vi "Otto_Stephen.vi"() -> ()   [LabVIEW 2020]
uses:
  <vilib>/MakerHub/LINX/Public/Peripherals/Analog/Analog Read 1 Chan.vi
  <vilib>/MakerHub/LINX/Public/Peripherals/Analog/Analog Read N Chans.vi
  <vilib>/MakerHub/LINX/Private/Local IO/LinxAnalogRead.vi
  <vilib>/MakerHub/LINX/Public/Utilities/Check Channel.vi
  <vilib>/MakerHub/LINX/Public/Utilities/Open Serial.vi
  <vilib>/MakerHub/LINX/Private/Utilties/Generate Error.vi
  <vilib>/MakerHub/LINX/LMH-LINX.lvlib
panel:
  out "Light":bool
  out "Voltage":dbl
  out "Waveform Chart":cluster{dbl, "f":dbl}(graph)
  in  "Offset":dbl
  in  "?":bool
  in  "Serial Port":refnum<visa-resource-name>="N/A"
  # "Stephen Otto\n011796499"
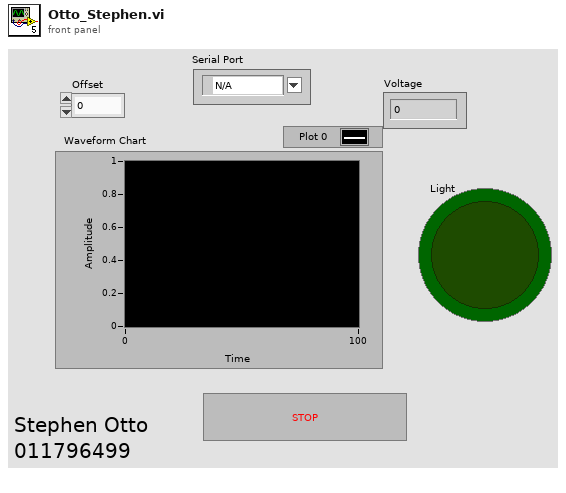
[diagram p1: front panel]
types:
  T1 = typedef "LMH-LINX.lvlib/LINX Ref.ctl" = cluster{"IO":T2, "Interface":T3, "LINX Device Config":T4}
  T2 = typedef "LMH-LINX.lvlib/Platform.ctl" = enum16{"Remote", "Local"}
  T3 = typedef "LMH-LINX.lvlib/Interface.ctl" = enum16{"Serial", "TCP"}
  T4 = typedef "LMH-LINX.lvlib/Device.lvlib/LINX Device Config.ctl" = cluster{"Interface":T3, "COM Port":refnum<visa-resource-name>, "TCP Configuration":T5, "Device Family":u8, "Device ID":u8, "Device Name":string, "TCP Ref":refnum<k5>, "Channels":T6}
  T5 = typedef "LMH-LINX.lvlib/Device.lvlib/TCP Config.ctl" = cluster{"IP Address":string, "Port":u16}
  T6 = typedef "LMH-LINX.lvlib/Channels.ctl" = cluster{"DI":u8[], "DO":u8[], "AI":u8[], "AO":u8[], "PWM":u8[], "QE":u8[], "UART":u8[], "I2C 2":u8[], "SPI":u8[], "CAN":u8[], "Servo":u8[], "AI Ref (V)":dbl, "AI Resolution (Bits)":u8, "AO Ref (V)":dbl, "AO Resolution (Bits)":u8}
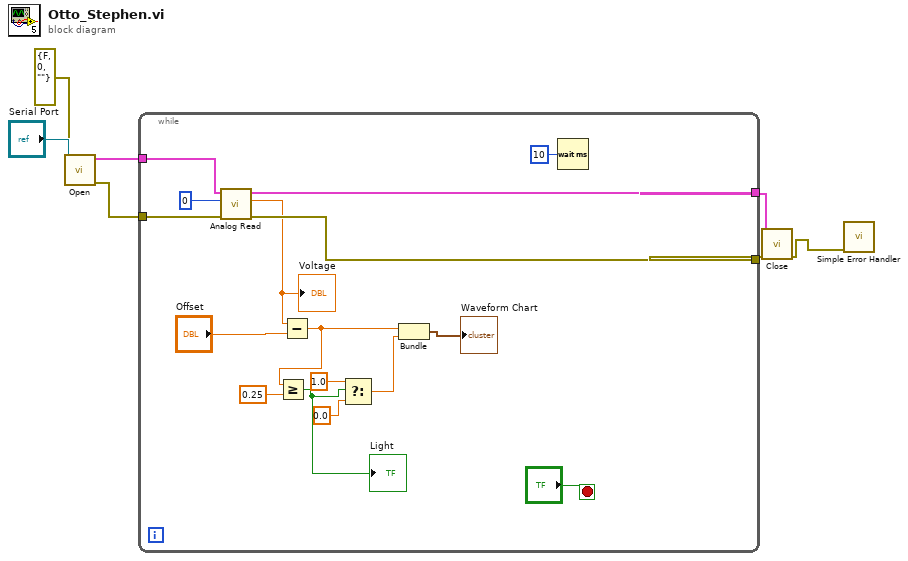
[diagram p0: block diagram]
diagram:
  n1 = call-poly <vilib>:"Open.vi"("Error In"=errorcluster {"status"=FALSE, "code"=0, "source"=""}, "Serial Port"="Serial Port") -> ("Error Out"=w3:errorcluster, "LINX Resource"=w6:T1)  [unwired: 7 in, 1 out]
  n2 = while {
    tunnel: [w23] -> w7
    tunnel: w6 -> [w22]
    tunnel: w3 -> [w20]
    tunnel: [w19] -> w2
    stop <- "?" stop-if-true
    n3 = call-poly <vilib>:"Analog Read.vi"("Error In"=w20, "Analog Channel"=u8 0, "LINX Resource"=w22) -> ("Error Out"=w19:errorcluster, "Voltage"=w15:dbl, "LINX Resource"=w23:T1)  [unwired: 5 in, 1 out]
    "Voltage" <- w15
    n4 = Subtract(x=w15, y="Offset") -> (x-y=w11:dbl)
    n5 = Greater Or Equal?(x=w11, y=0.25) -> (x >= y?=w8:bool)
    "Light" <- w8
    n6 = Select(t=1.0, s=w8, f=0.0) -> (s? t:f=w10:dbl)
    n7 = Bundle(w11, "f"=w10) -> (→"Waveform Chart":cluster{dbl, "f":dbl})  [unwired: 1 in]
    n8 = Wait (ms)(milliseconds to wait=u32 10) -> ()  [unwired: 1 out]
  }
  n9 = call <vilib>:"Close.vi"("Error In"=w2, "LINX Resource"=w7) -> ("Error Out"=w1:errorcluster)  [unwired: 9 in]
  n10 = call <vilib>:"Simple Error Handler.vi"("error in (no error)"=w1) -> ()  [unwired: 4 in, 5 out]
